vi "Get Project Item Reference.vi"(6 "Exclude dependencies (T)":bool=TRUE, 7 "TargetItem Refnum":refnum<vi>, 8 "error in (no error)":errorcluster, 9 "Type":string, 10 "Name":string, 11 "Project Refnum":refnum<vi>) -> (0 "error out":errorcluster, 2 "found?":bool, 3 "ProjectItem Refnum":refnum<vi>)   [LabVIEW 2015]
doc: "Retrieves a ProjectItem reference to an item (specified by name) under a specified TargetItem. If a TargetItem Refnum is not wired to this VI, then the My Computer target under the specified Project Refnum is used instead."
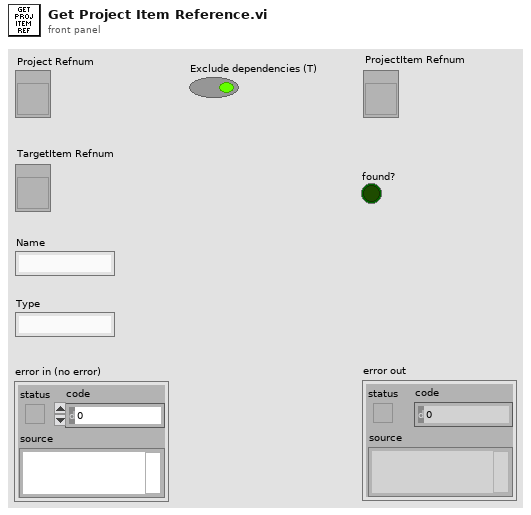
[diagram p1: front panel]
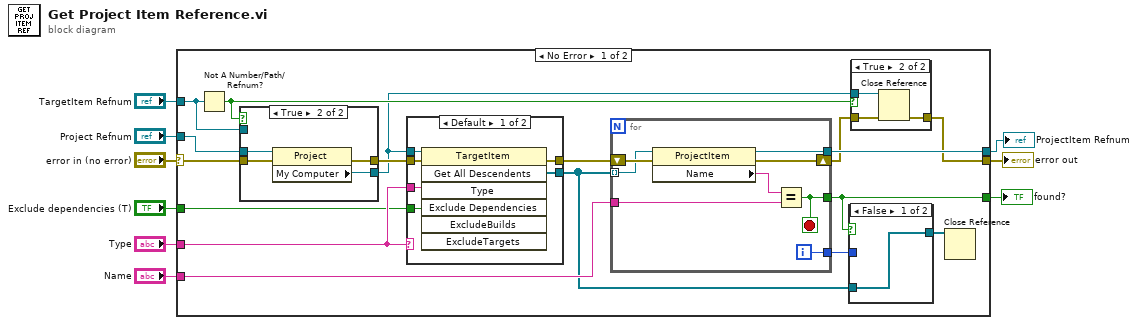
[diagram p0: block diagram]
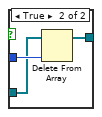
[diagram p2: hidden frame]
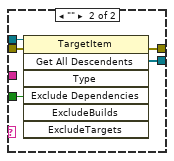
[diagram p4: hidden frame]
diagram:
  n1 = case shown="No Error" "error in (no error)" {
    selector: "error in (no error)" -> [w21 w60]
    tunnel: "Project Refnum" -> [w26 _]
    tunnel: "TargetItem Refnum" -> [w25 _]
    tunnel: [w10 w60] -> w7
    tunnel: [w22 _] -> w6
    tunnel: [w14 _] -> w5
    tunnel: "Name" -> [w20 _]
    tunnel: "Type" -> [w19 _]
    tunnel: "Exclude dependencies (T)" -> [w18 _]
    frame No Error {
      n2 = Not A Number/Path/Refnum?(number/path/refnum=w25) -> (NaN/Path/Refnum?=w17:bool)
      n3 = case shown="True" w17 {
        tunnel: [w55 w59] -> w16
        tunnel: [w54 w58] -> w23
        tunnel: w26 -> [_ w57]
        tunnel: w25 -> [w55 _]
        tunnel: w21 -> [w54 w56]
        frame False {
        }
        frame True {
          n4 = property class="Project"(reference=w57, error in=w56) -> (error out=w58:errorcluster, "My Computer"=w59:refnum<vi>)  [unwired: 1 out]
        }
      }
      n5 = case shown="Default" w19 {
        tunnel: [w40 w45] -> w24
        tunnel: w18 -> [w39 w44]
        tunnel: w16 -> [w38 w43]
        tunnel: [w37 w42] -> w12
        tunnel: w23 -> [w36 w41]
        tunnel: w19 -> [w35 _]
        frame Default {
          n6 = invoke class="TargetItem" method="Get All Descendents"(reference=w38, error in=w36, "Type"=w35, "Exclude Dependencies"=w39) -> (error out=w40:errorcluster, "All Descendents"=w37:refnum<vi>[])  [unwired: 3 in, 5 out]
        }
        frame "" {
          n7 = invoke class="TargetItem" method="Get All Descendents"(reference=w43, error in=w41, "Exclude Dependencies"=w44) -> (error out=w45:errorcluster, "All Descendents"=w42:refnum<vi>[])  [unwired: 4 in, 5 out]
        }
      }
      n8 = for {
        tunnel: w12 -> [w52] mode=indexing
        shift-right: [w51] -> w15
        shift-left: w24 -> [w53]
        tunnel: [w50] -> w22
        tunnel: w20 -> [w48]
        tunnel: [w47] -> w14
        tunnel: [w46] -> w13
        i -> [w46]
        stop <- w47 stop-if-true
        n9 = property class="ProjectItem"(reference=w52, error in=w53) -> (reference out=w50:refnum<vi>, error out=w51:errorcluster, "Name"=w49:string)
        n10 = Equal?(x=w49, y=w48) -> (x = y?=w47:bool)
      }
      n11 = case shown="False" w14 {
        tunnel: w13 -> [_ w30]
        tunnel: w12 -> [w27 w29]
        tunnel: [w27 w28] -> w11
        frame False {
        }
        frame True {
          n12 = Delete From Array(array=w29, index=w30) -> (array with subset deleted=w28:refnum<vi>[])  [unwired: 1 in, 1 out]
        }
      }
      n13 = case shown="True" w17 {
        tunnel: w15 -> [w31 w34]
        tunnel: w16 -> [_ w32]
        tunnel: [w31 w33] -> w10
        frame False {
        }
        frame True {
          n14 = Close Reference(reference=w32, error in (no error)=w34) -> (error out=w33:errorcluster)
        }
      }
      n15 = Close Reference(reference=w11) -> ()  [unwired: 1 in, 1 out]
    }
    frame Error {
    }
  }
  "ProjectItem Refnum" <- w6
  "error out" <- w7
  "found?" <- w5
